vi "Check if Timed Out).vi"(6 "Time out":dbl, 11 "Main Array in":T1={"FIFO Array"=[], "Dist (ft)"=0.0, "MaxSpeed (ft/s)"=0.0, "TimeOut (s)"=0.0, "Timer Value"=0, "DriveStraightDistance"=[], "ModuleTravelPosition"=[], "First Time"=FALSE, "Current Step"={"Auto States"=enum."Unknown", "Dist"=4.3, "Radians"=0.0, "MaxSpeed (ft/s)"=1.2, "TimeOut (s)"=10.0, "CMD"="", "ArmSetpoints"=enum."ShoulderRest"}}) -> (1 "Timed Out":bool, 3 "Main Array out":T1={"FIFO Array"=[], "Dist (ft)"=0.0, "MaxSpeed (ft/s)"=0.0, "TimeOut (s)"=0.0, "Timer Value"=0, "DriveStraightDistance"=[], "ModuleTravelPosition"=[], "First Time"=FALSE, "Current Step"={"Auto States"=enum."Unknown", "Dist"=4.3, "Radians"=0.0, "MaxSpeed (ft/s)"=1.2, "TimeOut (s)"=10.0, "CMD"="", "ArmSetpoints"=enum."ShoulderRest"}})   [LabVIEW 2023]
uses:
  Auton Main Array.ctl
  State Machine/FIFO Array.ctl
  State Machine/Auot FIFO.ctl
  State Machine/Auot States.ctl
  Shoulder/ShoulderGetSetpointEnum.ctl
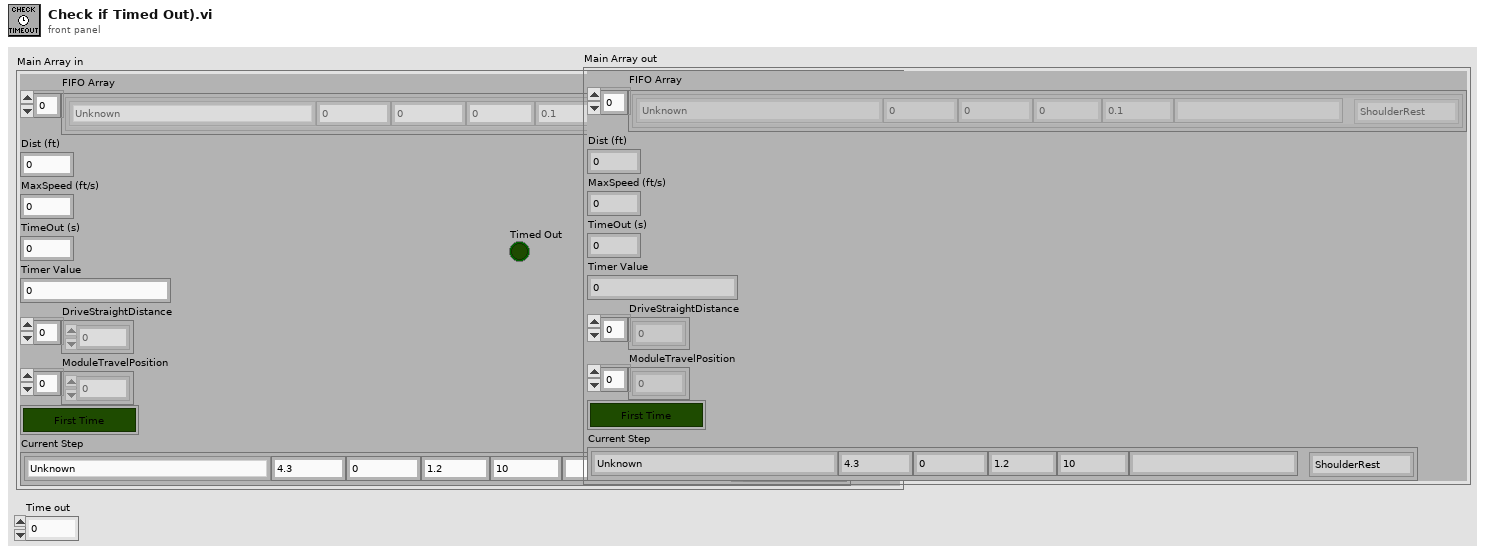
[diagram p1: front panel]
types:
  T1 = typedef "Auton Main Array.ctl" = cluster{"FIFO Array":T2, "Dist (ft)":dbl, "MaxSpeed (ft/s)":dbl, "TimeOut (s)":dbl, "Timer Value":u32, "DriveStraightDistance":dbl[], "ModuleTravelPosition":dbl[], "First Time":bool, "Current Step":T3}
  T2 = typedef "FIFO Array.ctl" = T3[]
  T3 = typedef "Auot FIFO.ctl" = cluster{"Auto States":T4, "Dist":dbl, "Radians":dbl, "MaxSpeed (ft/s)":dbl, "TimeOut (s)":dbl, "CMD":string, "ArmSetpoints":T5}
  T4 = typedef "Auot States.ctl" = enum16{"Unknown", "Initilize", "Intake", "Move Arm", "Drive Straight", "Drive Trajorctory", "Drive Turn", "Send Bool CMD", "Set Target", "Shoot", "Wait", "Exit"}
  T5 = typedef "ShoulderGetSetpointEnum.ctl" = enum16{"Select", "ShoulderRest", "ShoulderSpeaker", "ShoulderAmp"}
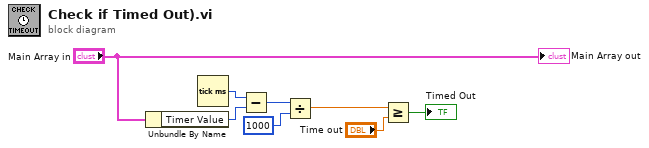
[diagram p0: block diagram]
diagram:
  n1 = Unbundle By Name("Main Array in") -> ("Timer Value"=w6:u32)
  n2 = Tick Count (ms)() -> (millisecond timer value=w5:u32)
  n3 = Subtract(x=w5, y=w6) -> (x-y=w7:u32)
  n4 = Divide(x=w7, y=u32 1000) -> (x/y=w4:dbl)
  n5 = Greater Or Equal?(x=w4, y="Time out") -> (x >= y?=→"Timed Out":bool)
  "Main Array out" <- "Main Array in"
